vi "Method.vi"(4 "Bool":refnum<class "Abs_U64 Integer.lvclass">) -> (1 "Result":T1)   [LabVIEW 2021, in "NOT_U64.lvclass"]
uses:
  NOT_U64.lvclass
  Abs_Types/U64 Integer/Abs_U64 Integer.lvclass
  Abs_Type.ctl
  C:/TSA/LV_Abstract/Source/Functions/Support/Function/One Terminal/U64/AbsFunc_One Term_U64.lvclass
  C:/Program Files (x86)/National Instruments/LabVIEW 2021/vi.lib/TSA/Abstract Data Classes/Abs_Types/U64 Integer/Abs_U64 Integer.lvclass
  Support/Function/One Terminal/U64/AbsFunc_One Term_U64.lvclass/AbsFunc_One Term_U64.ctl
  Support/Function/One Terminal/U64/Properties/Write Numeric A.vi
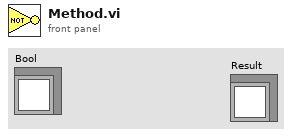
[diagram p1: front panel]
types:
  T1 = typedef "NOT_U64.lvclass/Abs_Type.ctl" = refnum<class "Abs_U64 Integer.lvclass">
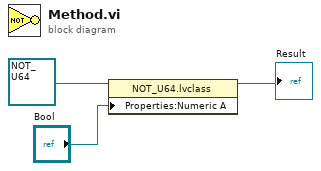
[diagram p0: block diagram]
diagram:
  n1 = property class="NOT_U64.lvclass"(reference=refnum<class "NOT_U64.lvclass"> refnum ("Functions.lvlib:Logic.lvlib:NOT.lvclass"), "Properties:Numeric A"="Bool") -> (reference out=→"Result":refnum<class "NOT_U64.lvclass">)  [unwired: 1 in, 1 out]
